vi "Time.vi"(8 "error in (no error)":errorcluster, 10 "Control In":T1={"I-O.lvclass"=refnum, "Motion.lvclass"=refnum, "Dispenser.lvclass"=refnum}, 11 "CAD Dispense2 in":refnum<class "CAD Dispense2.lvclass">) -> (0 "error out":errorcluster, 1 "Timing Data":i32[](array[numeric]), 2 "Control Out":T1, 3 "CAD Dispense2 out":refnum<class "CAD Dispense2.lvclass">)   [LabVIEW 2016, in "CAD Dispense2.lvclass"]
uses:
  CAD Dispense2.lvclass
  D:/UCSB-Gantry 0418/V5/Classes/Routine/Dispense/Dispense.lvclass
  Controller/Controllers.ctl
  Controller/I-O/I-O.lvclass
  Controller/Motion/A3200/A3200.lvclass
  Controller/Dispenser/Dispenser.lvclass
  Controller/Motion/Motion.lvclass
  CAD Dispense2.lvclass/CAD Dispense2.ctl
  Dispense.lvclass/Dispense.ctl
  Read Z Height.vi
  Read Z speed.vi
  Controller/Controller.lvclass
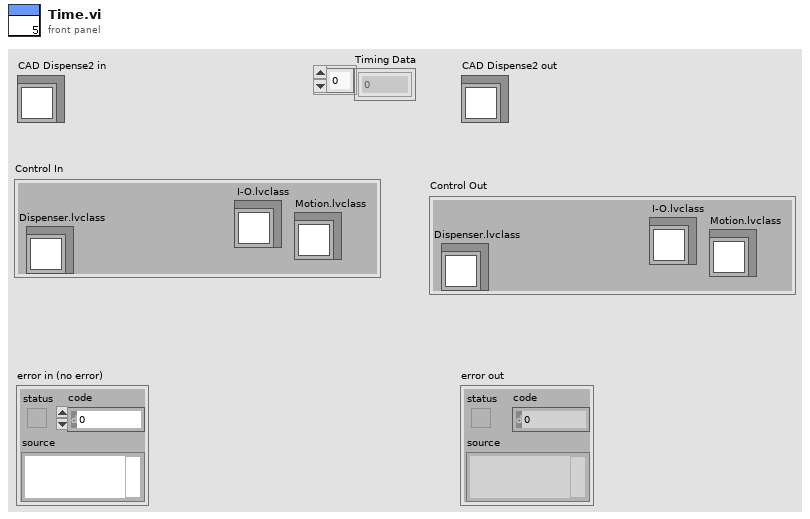
[diagram p1: front panel]
types:
  T1 = typedef "Controller.lvclass/Controllers.ctl" = cluster{"I-O.lvclass":refnum<class "I-O.lvclass">, "Motion.lvclass":refnum<class "Motion.lvclass">, "Dispenser.lvclass":refnum<class "Dispenser.lvclass">}
  T2 = cluster{"Endpoints":dbl[][], "Center":dbl[], "Dispense Type":enum16{"N-gon", "Square", "Arc", "Dot", "Line", "Circle"}, "CW/CCW":dbl}[]
  T3 = enum16{"N-gon", "Square", "Arc", "Dot", "Line", "Circle"}
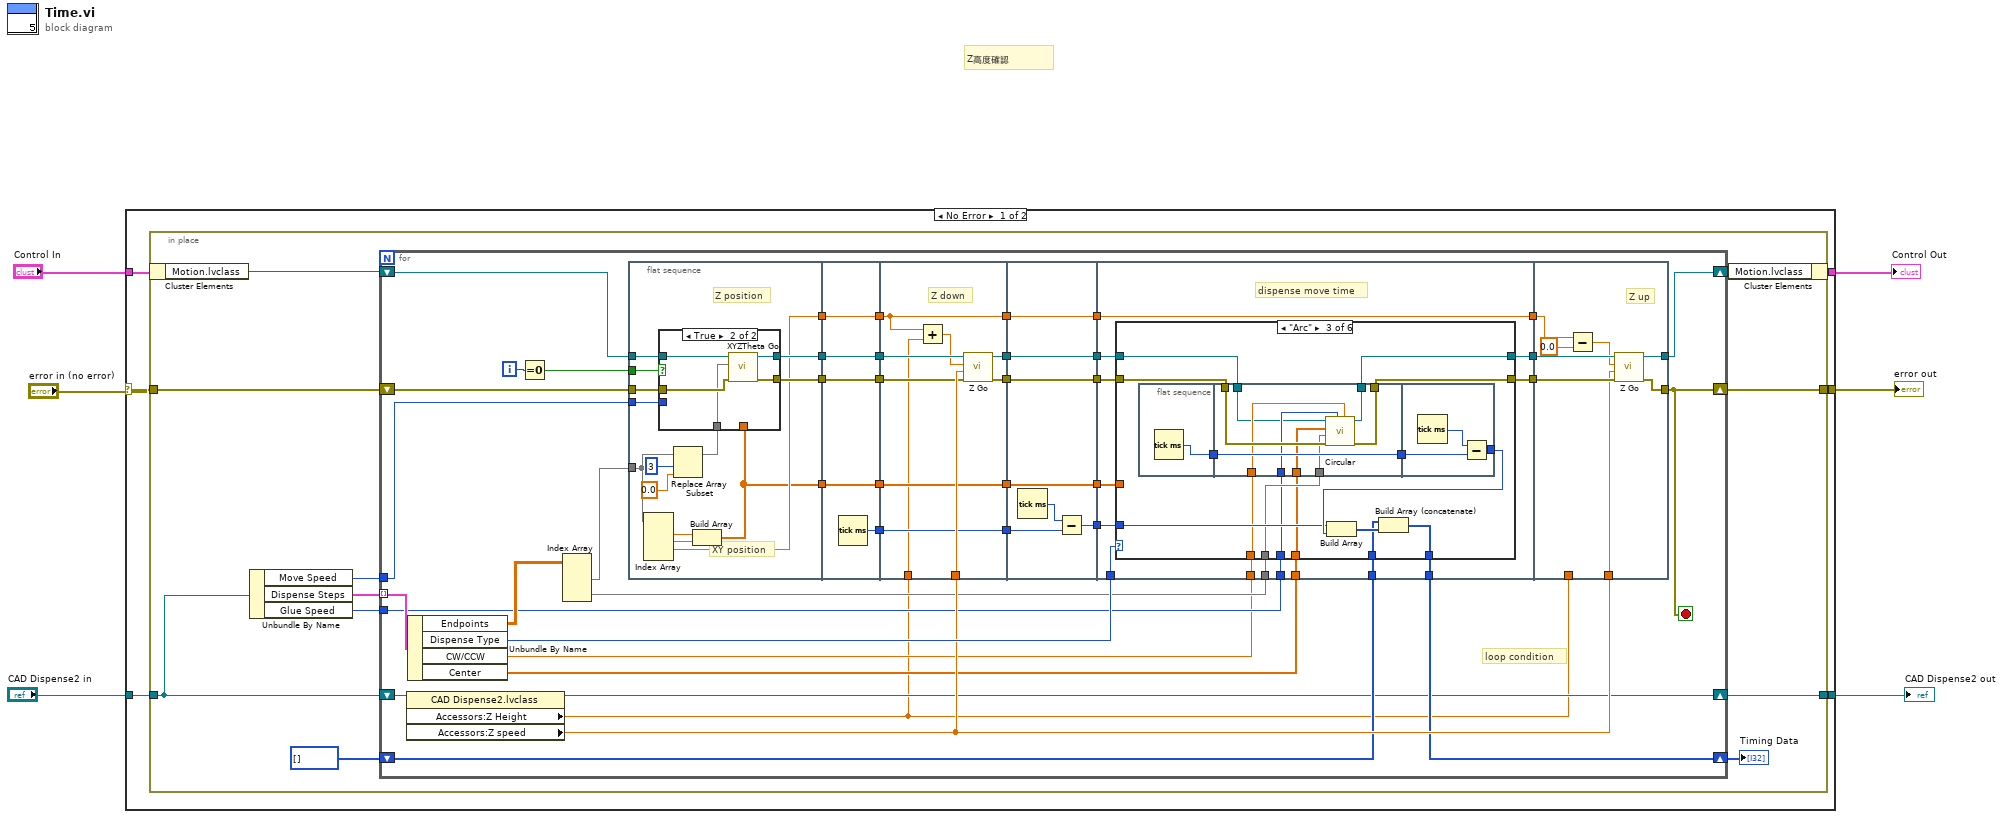
[diagram p0: block diagram]
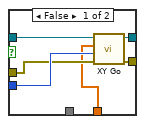
[diagram p2: hidden frame]
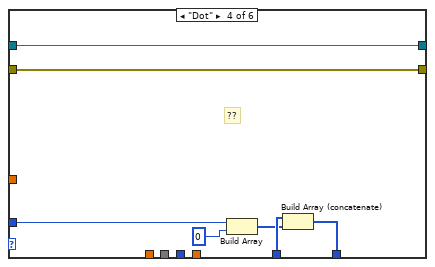
[diagram p5: hidden frame]
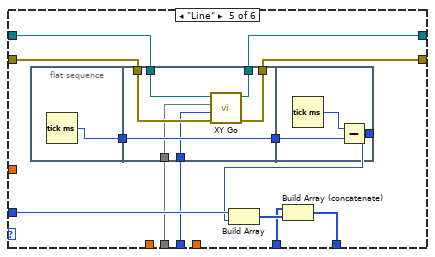
[diagram p6: hidden frame]
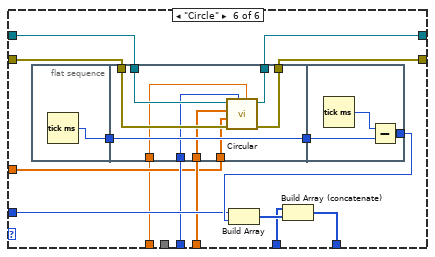
[diagram p7: hidden frame]
diagram:
  # "Z高度確認"
  n1 = case shown="No Error" "error in (no error)" {
    selector: "error in (no error)" -> [w10 w230]
    tunnel: "Control In" -> [w12 w231]
    tunnel: "CAD Dispense2 in" -> [w11 w229]
    tunnel: [w9 w231] -> w3
    tunnel: [w8 w230] -> w2
    tunnel: [w7 w229] -> w1
    frame No Error {
      n2 = in-place {
        in-place-border: w11 -> [w18]
        in-place-border: w10 -> [w21]
        in-place-border: [w14] -> w8
        in-place-border: [w13] -> w7
        n3 = in-place-cluster #1(w12) -> ("Motion.lvclass"=w20:refnum<class "Motion.lvclass">)
        n4 = Unbundle By Name(w18) -> ("Move Speed"=w16:i32, "Dispense Steps"=w17:T2, "Glue Speed"=w15:i32)
        n5 = for {
          shift-right: [w38] -> w22
          shift-left: i32[] [] ("Timing Data") -> [w37]
          shift-right: [w33] -> w19
          shift-left: w20 -> [w60]
          tunnel: w17 -> [w65] mode=indexing
          tunnel: w16 -> [w61]
          tunnel: w15 -> [w35]
          shift-right: [w25] -> w14
          shift-left: w21 -> [w55]
          shift-right: [w32] -> w13
          shift-left: w18 -> [w66]
          i -> [w64]
          stop <- w25 stop-if-true
          # "loop condition"
          n6 = property class="CAD Dispense2.lvclass"(reference=w66) -> (reference out=w32:refnum<class "CAD Dispense2.lvclass">, "Accessors:Z Height"=w24:dbl, "Accessors:Z speed"=w39:dbl)  [unwired: 1 in, 1 out]
          n7 = Unbundle By Name(w65) -> ("Endpoints"=w62:dbl[][], "Dispense Type"=w50:T3, "CW/CCW"=w26:dbl, "Center"=w27:dbl[])
          n8 = Equal To 0?(x=w64) -> (x = 0?=w63:bool)
          n9 = Index Array(array=w62) -> (element #1=w34:dbl[], element #2=w36:dbl[])  [unwired: 4 in]
          n10 = flat-sequence {
            tunnel: w63 -> [w80]
            tunnel: w61 -> [w79]
            tunnel: w60 -> [w78]
            tunnel: [w77] -> w59
            tunnel: [w72] -> w56
            tunnel: w55 -> [w76]
            tunnel: [w75] -> w53
            tunnel: w34 -> [w68]
            tunnel: [w71] -> w31
            tunnel: w59 -> [w96]
            tunnel: [w96] -> w58
            tunnel: [w95] -> w57
            tunnel: w56 -> [w95]
            tunnel: [w94] -> w54
            tunnel: w53 -> [w94]
            tunnel: [w93] -> w52
            tunnel: w31 -> [w92]
            tunnel: [w92] -> w30
            tunnel: w24 -> [w97]
            tunnel: w58 -> [w106]
            tunnel: w57 -> [w99]
            tunnel: w39 -> [w104]
            tunnel: w54 -> [w103]
            tunnel: w52 -> [w102]
            tunnel: [w102] -> w51
            tunnel: [w101] -> w47
            tunnel: [w100] -> w45
            tunnel: [w99] -> w42
            tunnel: w30 -> [w98]
            tunnel: [w98] -> w29
            tunnel: w51 -> [w112]
            tunnel: [w111] -> w49
            tunnel: [w110] -> w48
            tunnel: w47 -> [w110]
            tunnel: [w109] -> w46
            tunnel: w45 -> [w109]
            tunnel: w42 -> [w108]
            tunnel: [w108] -> w41
            tunnel: w29 -> [w107]
            tunnel: [w107] -> w28
            tunnel: w50 -> [w127]
            tunnel: w49 -> [w126]
            tunnel: w48 -> [w125]
            tunnel: w46 -> [w124]
            tunnel: [w123] -> w44
            tunnel: [w122] -> w43
            tunnel: w41 -> [w121]
            tunnel: [w121] -> w40
            tunnel: [w120] -> w38
            tunnel: w37 -> [w119]
            tunnel: w36 -> [w118]
            tunnel: w35 -> [w117]
            tunnel: w27 -> [w116]
            tunnel: w28 -> [w115]
            tunnel: w26 -> [w114]
            tunnel: w44 -> [w228]
            tunnel: w43 -> [w227]
            tunnel: w40 -> [w223]
            tunnel: w39 -> [w226]
            tunnel: [w225] -> w33
            tunnel: [w224] -> w25
            tunnel: w24 -> [_]
            frame #0 {
              # "XY position"
              # "Z position"
              n11 = Index Array(array=w68) -> (element #1=w74:dbl, element #2=w73:dbl, element #3=w72:dbl)  [unwired: 4 in, 1 out]
              n12 = Replace Array Subset(array=w68, new element=0.0 ("new element/subarray"), index=3) -> (w69:dbl[])
              n13 = Build Array(w74, w73) -> (w71:dbl[])
              n14 = case shown="True" w80 {
                tunnel: w79 -> [w86 _]
                tunnel: w78 -> [w85 w91]
                tunnel: [w84 w90] -> w77
                tunnel: w76 -> [w83 w89]
                tunnel: [w82 w88] -> w75
                tunnel: w71 -> [w81 _]
                tunnel: w69 -> [_ w87]
                frame False {
                  n15 = call-dynamic "XY Go.vi"("error in (no error)"=w83, "Speed"=w86, "XY"=w81, "Motion in"=w85) -> ("error out"=w82:errorcluster, "Motion out"=w84:refnum<class "Motion.lvclass">)  [unwired: 6 in]
                }
                frame True {
                  n16 = call "XYZTheta Go.vi"("error in (no error)"=w89, "XYZTheta In"=w87, "Motion in"=w91) -> ("error out"=w88:errorcluster, "Motion out"=w90:refnum<class "Motion.lvclass">)  [unwired: 6 in, 1 out]
                }
              }
            }
            frame #1 {
              n17 = Tick Count (ms)() -> (millisecond timer value=w93:u32)
            }
            frame #2 {
              # "Z down"
              n18 = Add(x=w99, y=w97) -> (x+y=w105:dbl)
              n19 = call-dynamic "Z Go.vi"("error in (no error)"=w103, "Speed"=w104, "Position"=w105, "Motion in"=w106) -> ("error out"=w101:errorcluster, "Motion out"=w100:refnum<class "Motion.lvclass">)  [unwired: 6 in]
            }
            frame #3 {
              n20 = Tick Count (ms)() -> (millisecond timer value=w113:u32)
              n21 = Subtract(x=w113, y=w112) -> (x-y=w111:u32)
            }
            frame #4 {
              # "dispense move time"
              n22 = case shown="\"Arc\"" w127 {
                tunnel: w126 -> [_ _ w142 w166 w174 w201]
                tunnel: w125 -> [w129 w132 w135 w167 w179 w198]
                tunnel: w124 -> [w130 w133 w137 w168 w181 w200]
                tunnel: [w130 w133 w136 w168 w180 w199] -> w123
                tunnel: [w129 w132 w134 w167 w178 w197] -> w122
                tunnel: [w128 w131 w144 w162 w171 w203] -> w120
                tunnel: w119 -> [w128 w131 w143 w164 w172 w202]
                tunnel: w118 -> [_ _ w141 _ w170 _]
                tunnel: w117 -> [_ _ w139 _ w169 w196]
                tunnel: w116 -> [_ _ w140 _ _ w195]
                tunnel: w115 -> [_ _ _ _ _ w194]
                tunnel: w114 -> [_ _ w138 _ _ w193]
                frame "N-gon", Default {
                }
                frame "Square" {
                }
                frame "Arc" {
                  n23 = flat-sequence {
                    tunnel: [w149] -> w148
                    tunnel: w137 -> [w150]
                    tunnel: [w155] -> w136
                    tunnel: w135 -> [w156]
                    tunnel: [w157] -> w134
                    tunnel: w148 -> [w158]
                    tunnel: [w158] -> w147
                    tunnel: w139 -> [w154]
                    tunnel: w140 -> [w153]
                    tunnel: w141 -> [w152]
                    tunnel: w138 -> [w151]
                    tunnel: w147 -> [w160]
                    tunnel: [w159] -> w145
                    frame #0 {
                      n24 = Tick Count (ms)() -> (millisecond timer value=w149:u32)
                    }
                    frame #1 {
                      n25 = call-dynamic "Circular.vi"("Direction"=w151, "Speed"=w154, "error in (no error)"=w156, "XY End"=w152, "XY Center"=w153, "Motion in"=w150) -> ("error out"=w157:errorcluster, "Motion out"=w155:refnum<class "Motion.lvclass">)  [unwired: 4 in]
                    }
                    frame #2 {
                      n26 = Tick Count (ms)() -> (millisecond timer value=w161:u32)
                      n27 = Subtract(x=w161, y=w160) -> (x-y=w159:u32)
                    }
                  }
                  n28 = Build Array(w142, w145) -> (w146:u32[])
                  n29 = Build Array (concatenate)(w143, w146) -> (w144:u32[])
                }
                frame "Dot" {
                  # "??"
                  n30 = Build Array(w166, u32 0 ("element")) -> (w163:u32[])
                  n31 = Build Array (concatenate)(w164, w163) -> (w162:u32[])
                }
                frame "Line" {
                  n32 = flat-sequence {
                    tunnel: [w182] -> w177
                    tunnel: w181 -> [w189]
                    tunnel: [w188] -> w180
                    tunnel: w179 -> [w187]
                    tunnel: [w186] -> w178
                    tunnel: w177 -> [w185]
                    tunnel: [w185] -> w176
                    tunnel: w170 -> [w184]
                    tunnel: w169 -> [w183]
                    tunnel: w176 -> [w191]
                    tunnel: [w190] -> w173
                    frame #0 {
                      n33 = Tick Count (ms)() -> (millisecond timer value=w182:u32)
                    }
                    frame #1 {
                      n34 = call-dynamic "XY Go.vi"("error in (no error)"=w187, "Speed"=w183, "XY"=w184, "Motion in"=w189) -> ("error out"=w186:errorcluster, "Motion out"=w188:refnum<class "Motion.lvclass">)  [unwired: 6 in]
                    }
                    frame #2 {
                      n35 = Tick Count (ms)() -> (millisecond timer value=w192:u32)
                      n36 = Subtract(x=w192, y=w191) -> (x-y=w190:u32)
                    }
                  }
                  n37 = Build Array(w174, w173) -> (w175:u32[])
                  n38 = Build Array (concatenate)(w172, w175) -> (w171:u32[])
                }
                frame "Circle" {
                  n39 = flat-sequence {
                    tunnel: [w208] -> w207
                    tunnel: w200 -> [w214]
                    tunnel: [w213] -> w199
                    tunnel: w198 -> [w215]
                    tunnel: [w216] -> w197
                    tunnel: w207 -> [w217]
                    tunnel: [w217] -> w206
                    tunnel: w196 -> [w212]
                    tunnel: w195 -> [w211]
                    tunnel: w194 -> [w210]
                    tunnel: w193 -> [w209]
                    tunnel: w206 -> [w219]
                    tunnel: [w218] -> w204
                    frame #0 {
                      n40 = Tick Count (ms)() -> (millisecond timer value=w208:u32)
                    }
                    frame #1 {
                      n41 = call-dynamic "Circular.vi"("Direction"=w209, "Speed"=w212, "error in (no error)"=w215, "XY End"=w210, "XY Center"=w211, "Motion in"=w214) -> ("error out"=w216:errorcluster, "Motion out"=w213:refnum<class "Motion.lvclass">)  [unwired: 4 in]
                    }
                    frame #2 {
                      n42 = Tick Count (ms)() -> (millisecond timer value=w220:u32)
                      n43 = Subtract(x=w220, y=w219) -> (x-y=w218:u32)
                    }
                  }
                  n44 = Build Array(w201, w204) -> (w205:u32[])
                  n45 = Build Array (concatenate)(w202, w205) -> (w203:u32[])
                }
              }
            }
            frame #5 {
              # "Z up"
              n46 = Subtract(x=w223, y=0.0) -> (x-y=w222:dbl)
              n47 = call-dynamic "Z Go.vi"("error in (no error)"=w227, "Speed"=w226, "Position"=w222, "Motion in"=w228) -> ("error out"=w224:errorcluster, "Motion out"=w225:refnum<class "Motion.lvclass">)  [unwired: 6 in]
            }
          }
        }
        "Timing Data" <- w22
        n48 = in-place-cluster #1("Motion.lvclass"=w19) -> (w9:T1)
      }
    }
    frame Error {
    }
  }
  "error out" <- w2
  "CAD Dispense2 out" <- w1
  "Control Out" <- w3
